vi "Curve Fit.vi"(7 "error in (no error)":errorcluster, 10 "Graph Data In":T1) -> (0 "error out":errorcluster, 2 "New Graph Data Out":T1)   [LabVIEW 2013, in "Diode Characterization.lvlib" / "Diode IV.lvclass"]
doc: "Finds the best fit exponential curve for each waveform in Data In. The graph data out consists of a plot of the best fit curve and an annotation describing the parameters and residual value."
uses:
  Diode IV.lvclass
  graphdata.ctl
  <vilib>/Utility/miscctls.llb/LVAnnotationListTypeDef.ctl
  <vilib>/Utility/miscctls.llb/LVCursorListTypeDef.ctl
  <vilib>/Analysis/NI_AALPro.lvlib
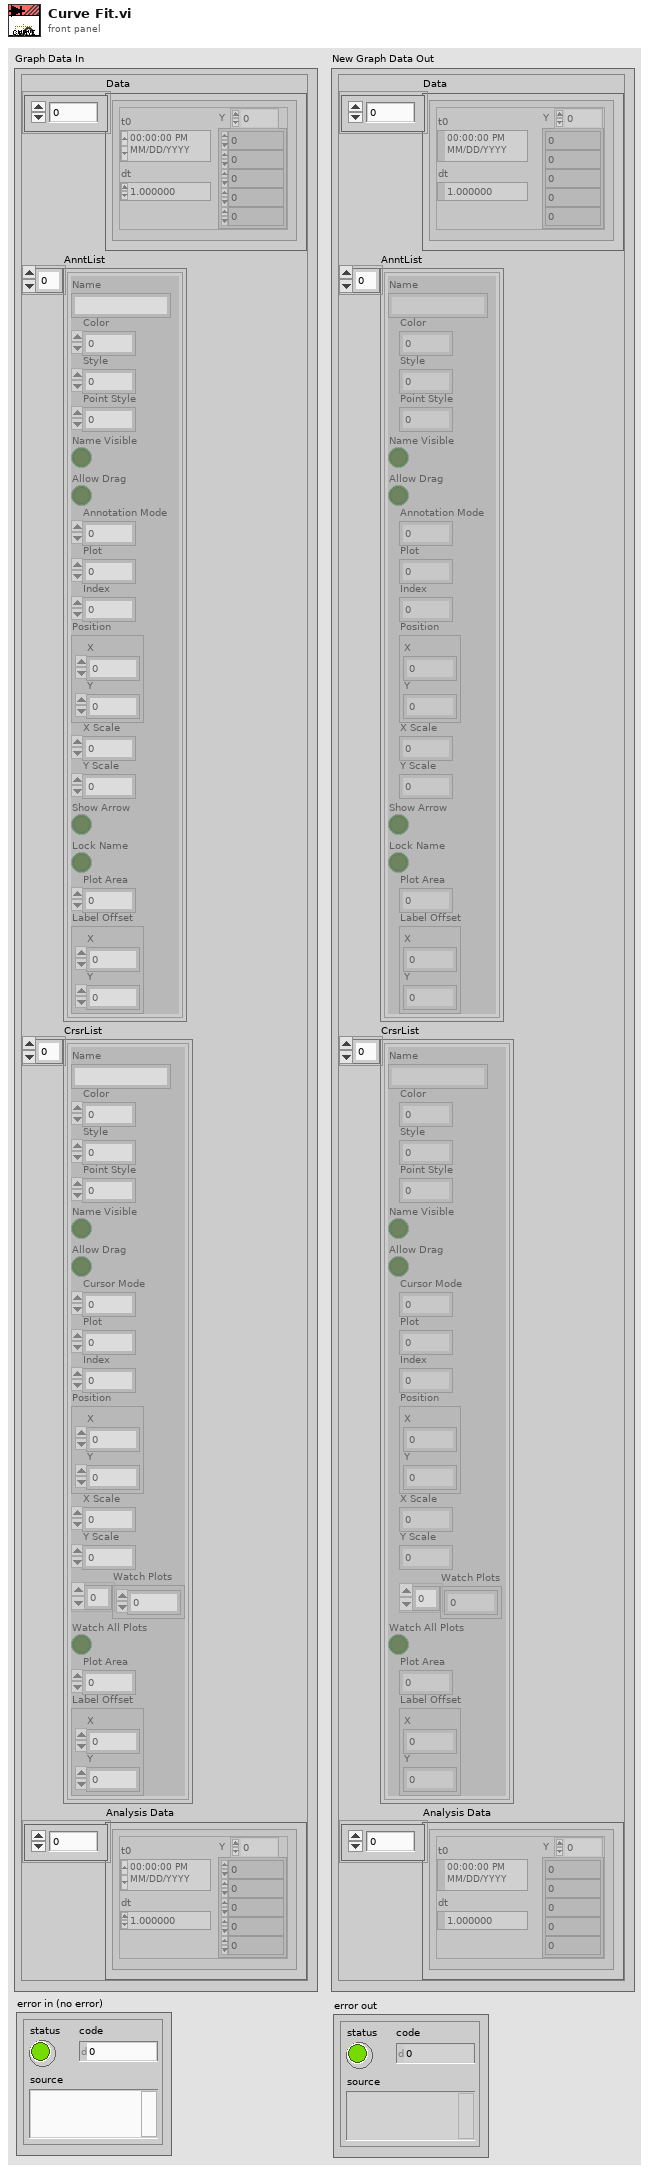
[diagram p1: front panel]
types:
  T1 = typedef "Diode Characterization.lvlib/Diode IV.lvclass/graphdata.ctl" = cluster{"Data":waveform(dbl)[], "AnntList":T2, "CrsrList":T3, "Analysis Data":waveform(dbl)[]}
  T2 = typedef "LVAnnotationListTypeDef.ctl" = cluster{"Name":string, "Color":u32, "Style":u8, "Point Style":u8, "Name Visible":bool, "Allow Drag":bool, "Annotation Mode":u32, "Plot":i32, "Index":i32, "Position":cluster{"X":dbl, "Y":dbl}, "X Scale":u32, "Y Scale":u32, "Show Arrow":bool, "Lock Name":bool, "Plot Area":i32, "Label Offset":cluster{"X":dbl, "Y":dbl}}[]
  T3 = typedef "LVCursorListTypeDef.ctl" = cluster{"Name":string, "Color":u32, "Style":u8, "Point Style":u8, "Name Visible":bool, "Allow Drag":bool, "Cursor Mode":u32, "Plot":i32, "Index":i32, "Position":cluster{"X":dbl, "Y":dbl}, "X Scale":u32, "Y Scale":u32, "Watch Plots":i32[], "Watch All Plots":bool, "Plot Area":i32, "Label Offset":cluster{"X":dbl, "Y":dbl}}[]
  T4 = cluster{"Name":string, "Color":u32, "Style":u8, "Point Style":u8, "Name Visible":bool, "Allow Drag":bool, "Annotation Mode":u32, "Plot":i32, "Index":i32, "Position":cluster{"X":dbl, "Y":dbl}, "X Scale":u32, "Y Scale":u32, "Show Arrow":bool, "Lock Name":bool, "Plot Area":i32, "Label Offset":cluster{"X":dbl, "Y":dbl}}
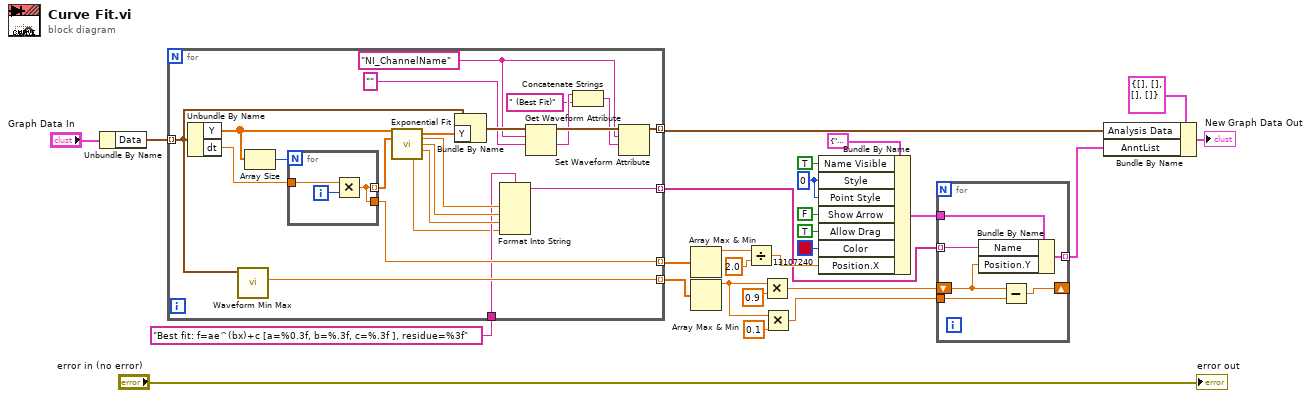
[diagram p0: block diagram]
diagram:
  w19 = u8 0 ("Style")
  n1 = Unbundle By Name("Graph Data In") -> ("Data"=w15:waveform(dbl)[])
  n2 = for {
    tunnel: w15 -> [w35] mode=indexing
    tunnel: [w41] -> w23 mode=indexing
    tunnel: [w34] -> w13 mode=indexing
    tunnel: [w33] -> w14 mode=indexing
    tunnel: "Best fit: f=ae^(bx)+c [a=%0.3f, b=%.3f, c=%.3f ], residue=%3f" ("format string") -> [w29]
    tunnel: [w28] -> w3 mode=indexing
    w39 = "NI_ChannelName" ("name")
    n3 = Unbundle By Name(w35) -> ("Y"=w45:dbl[], "dt"=w47:dbl)
    n4 = call <vilib>:"Waveform Min Max.vi"("waveform in"=w35) -> ("Y max"=w34:dbl)  [unwired: 5 in, 5 out]
    n5 = Array Size(array=w45) -> (size(s)=w48:i32)
    n6 = for {
      N: w48 -> [_]
      tunnel: w47 -> [w50]
      tunnel: [w49] -> w46 mode=indexing
      tunnel: [w49] -> w33
      i -> [w51]
      n7 = Multiply(x=w50, y=w51) -> (x*y=w49:dbl)
    }
    n8 = call <vilib>:"Exponential Fit.vi"("Y"=w45, "X"=w46) -> ("Best Exponential Fit"=w44:dbl[], "amplitude"=w32:dbl, "damping"=w31:dbl, "offset"=w30:dbl, "residue"=w27:dbl)  [unwired: 8 in, 1 out]
    n9 = Bundle By Name(cluster=w35, "Y"=w44) -> (w43:waveform(dbl))
    n10 = Format Into String(format string=w29, w32, w31, w30, w27) -> (resulting string=w28:string)  [unwired: 2 in, 1 out]
    n11 = Get Waveform Attribute(5:"" ("name"), 6:w39, 7:w43) -> (1:w38:string, 3:w42:waveform(dbl))  [unwired: 1 in, 2 out]
    n12 = Concatenate Strings(w38, " (Best Fit)" ("string")) -> (w36:string)
    n13 = Set Waveform Attribute(5:w36, 6:w39, 7:w42) -> (3:w41:waveform(dbl))  [unwired: 1 in, 2 out]
  }
  n14 = Array Max & Min(array=w14) -> (max value=w11:dbl)  [unwired: 3 out]
  n15 = Array Max & Min(array=w13) -> (max value=w5:dbl)  [unwired: 3 out]
  n16 = Divide(x=w11, y=2.0) -> (x/y=w9:dbl)
  n17 = Multiply(x=w5, y=0.9) -> (x*y=w7:dbl)
  n18 = Multiply(x=w5, y=0.1) -> (x*y=w6:dbl)
  n19 = Bundle By Name(cluster=T4 {"Name"="", "Color"=0, "Style"=0, "Point Style"=0, "Name Visible"=FALSE, "Allow Drag"=FALSE, "Annotation Mode"=0, "Plot"=0, "Index"=0, "Position"={"X"=0.0, "Y"=0.0}, "X Scale"=0, "Y Scale"=0, "Show Arrow"=FALSE, "Lock Name"=FALSE, "Plot Area"=0, "Label Offset"={"X"=0.0, "Y"=0.0}} ("element"), "Name Visible"=TRUE, "Style"=w19, "Point Style"=w19, "Show Arrow"=FALSE, "Allow Drag"=TRUE, "Color"=u32 13107240, "Position.X"=w9) -> (w12:T4)
  n20 = for {
    tunnel: w12 -> [w57]
    shift-right: [w54] -> _
    shift-left: w7 -> [w56]
    tunnel: w6 -> [w55]
    tunnel: [w53] -> w2 mode=indexing
    tunnel: w3 -> [w52] mode=indexing
    n21 = Bundle By Name(cluster=w57, "Name"=w52, "Position.Y"=w56) -> (w53:T4)
    n22 = Subtract(x=w56, y=w55) -> (x-y=w54:dbl)
  }
  n23 = Bundle By Name(cluster=T1 {"Data"=[], "AnntList"=[], "CrsrList"=[], "Analysis Data"=[]} ("Graph Data In"), "Analysis Data"=w23, "AnntList"=w2) -> (→"New Graph Data Out":T1)
  "error out" <- "error in (no error)"
